vi "Binary Number Mantissa and Exponent (U32).vi"(7 "Binary Number":u32 format="%.0b", 9 "Input Valid":bool=TRUE) -> (6 "Exponent (-N)":i8, 8 "Mantissa (M)":u32 format="%.0b", 10 "Output Valid":bool=TRUE)   [LabVIEW 2011]
doc: "This VI computes Mantissa and Exponent of Fixed Point Number\n\n<b> Latency = 4 Ticks </b>"
uses:
  <vilib>/rvi/FXPMathLib/basic elements/FxpDiscreteDelay/XNode/nifxpmath_DiscreteDelay.xnode
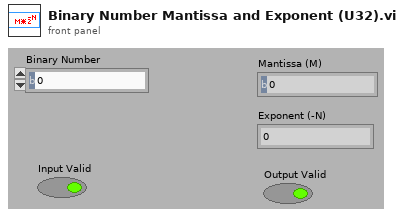
[diagram p1: front panel]
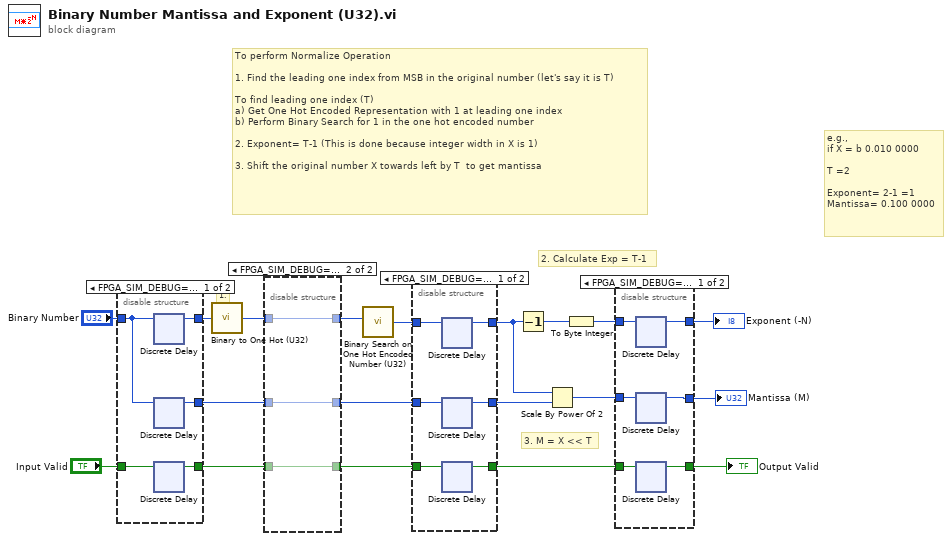
[diagram p0: block diagram]
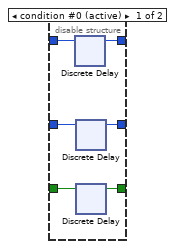
[diagram p4: hidden frame]
diagram:
  # "e.g.,\nif X = b 0.010 0000\n\nT =2\n\nExponent= 2-1 =1 \nMantissa= 0.100 0000"
  # "3. M = X << T"
  # "2. Calculate Exp = T-1"
  # "1."
  # "To perform Normalize Operation\n\n1. Find the leading one index from MSB in the original number (let's say it is T)\n\nTo find leading one index (T) \na) Get One Hot Encoded Representation with 1 at leading one index\nb) Perform Binary Search for 1 in the one hot encoded number\n\n2. Exponent= T-1 (This is done because integer width in X is 1)\n\n3. Shift the original number X towards left by T  to get mantissa"
  n1 = disable-structure shown="FPGA_SIM_DEBUG==FALSE, default" {
    disable-tunnel: [w24 w25] -> w14
    disable-tunnel: "Input Valid" -> [w23 w26]
    disable-tunnel: [w22 w26] -> w12
    disable-tunnel: [w21 w25] -> w6
    disable-tunnel: "Binary Number" -> [w20 w25]
    frame condition #0 (active) {
      n2 = xnode "Discrete Delay"("D"=w20) -> ("Q"=w24:u32)
      n3 = xnode "Discrete Delay"("D"=w20) -> ("Q"=w21:u32)
      n4 = xnode "Discrete Delay"("D"=w23) -> ("Q"=w22:bool)
    }
    frame condition #1 {
    }
  }
  n5 = call <userlib>:"Binary to One Hot (U32).vi"("Binary Number"=w14) -> ("One Hot Encoded Number"=w8:u32)  [unwired: 14 in]
  n6 = disable-structure shown="FPGA_SIM_DEBUG==TRUE" {
    disable-tunnel: w12 -> [w32 w33]
    disable-tunnel: [w31 w33] -> w10
    disable-tunnel: w8 -> [w30 w35]
    disable-tunnel: [w29 w35] -> w7
    disable-tunnel: w6 -> [w28 w34]
    disable-tunnel: [w27 w34] -> w3
    frame condition #0 (active) {
      n7 = xnode "Discrete Delay"("D"=w30) -> ("Q"=w29:u32)
      n8 = xnode "Discrete Delay"("D"=w28) -> ("Q"=w27:u32)
      n9 = xnode "Discrete Delay"("D"=w32) -> ("Q"=w31:bool)
    }
    frame condition #1 {
    }
  }
  n10 = call <userlib>:"Binary Search on One Hot Encoded Number (U32).vi"("One Hot Encoded Number"=w7) -> ("Binary Number"=w4:u8)  [unwired: 14 in]
  n11 = disable-structure shown="FPGA_SIM_DEBUG==FALSE, default" {
    disable-tunnel: [w41 w44] -> w18
    disable-tunnel: [w40 w43] -> w17
    disable-tunnel: [w39 w42] -> w11
    disable-tunnel: w10 -> [w38 w42]
    disable-tunnel: w4 -> [w37 w44]
    disable-tunnel: w3 -> [w36 w43]
    frame condition #0 (active) {
      n12 = xnode "Discrete Delay"("D"=w37) -> ("Q"=w41:u8)
      n13 = xnode "Discrete Delay"("D"=w36) -> ("Q"=w40:u32)
      n14 = xnode "Discrete Delay"("D"=w38) -> ("Q"=w39:bool)
    }
    frame condition #1 {
    }
  }
  n15 = Decrement(x=w18) -> (x-1=w19:u8)
  n16 = Scale By Power Of 2(n=w18, x=w17) -> (x*2^n=w1:u32)
  n17 = To Byte Integer(number=w19) -> (8bit integer=w2:i8)
  n18 = disable-structure shown="FPGA_SIM_DEBUG==FALSE, default" {
    disable-tunnel: [w50 w53] -> w16
    disable-tunnel: [w49 w52] -> w15
    disable-tunnel: w11 -> [w48 w51]
    disable-tunnel: [w47 w51] -> w9
    disable-tunnel: w2 -> [w46 w53]
    disable-tunnel: w1 -> [w45 w52]
    frame condition #0 (active) {
      n19 = xnode "Discrete Delay"("D"=w46) -> ("Q"=w50:i8)
      n20 = xnode "Discrete Delay"("D"=w45) -> ("Q"=w49:u32)
      n21 = xnode "Discrete Delay"("D"=w48) -> ("Q"=w47:bool)
    }
    frame condition #1 {
    }
  }
  "Mantissa (M)" <- w15
  "Exponent (-N)" <- w16
  "Output Valid" <- w9
